vi "Configure Video Trigger.vi"(0 "VISA resource name":refnum<visa-resource-name>, 1 "Wide Video Frequency Width (800E6 Hz)":dbl=800000000.0 format="%^#_9g", 2 "Narrow Video Frequency Center (1E9 Hz)":dbl=1000000000.0 format="%^#_9g", 5 "Minimum Power Level (-20 dB)":i32=-20 format="%^#_9g", 7 "Wide Video Mode (0: In)":u16(ring) items=["In", "Out", "Positive", "Negative"], 9 "Wide Video Frequency Center (1E9 Hz)":dbl=1000000000.0 format="%^#_9g", 11 "error in (no error)":errorcluster, 12 "Narrow Video Mode (0: In)":u16(ring) items=["In", "Out", "Positive", "Negative"], 13 "Narrow Video Frequency Width (13.8E6 Hz)":dbl=13800000.0 format="%^#_9g") -> (4 "VISA resource name out":refnum<visa-resource-name>, 15 "error out":errorcluster)   [LabVIEW 2011, in "Agilent E5052X.lvlib"]
doc: "Configure the video trigger settings for Transient Measurements. \n\n<b>Note: </b>\n\n Be sure to set this first before setting the trigger source to one of the video modes."
uses:
  Agilent E5052X.lvlib
panel:
  # "Wideband Settings"
  # "Narrowband Settings"
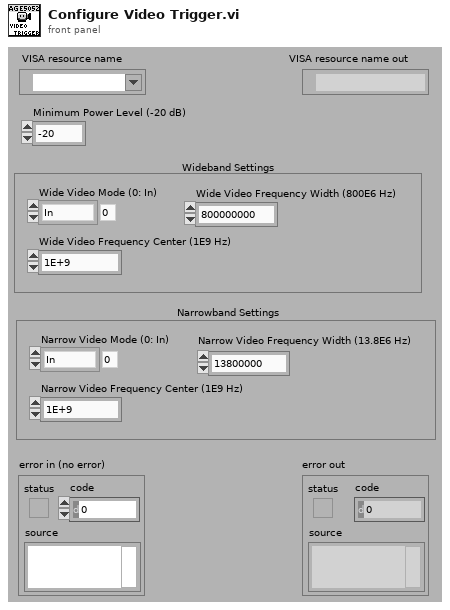
[diagram p1: front panel]
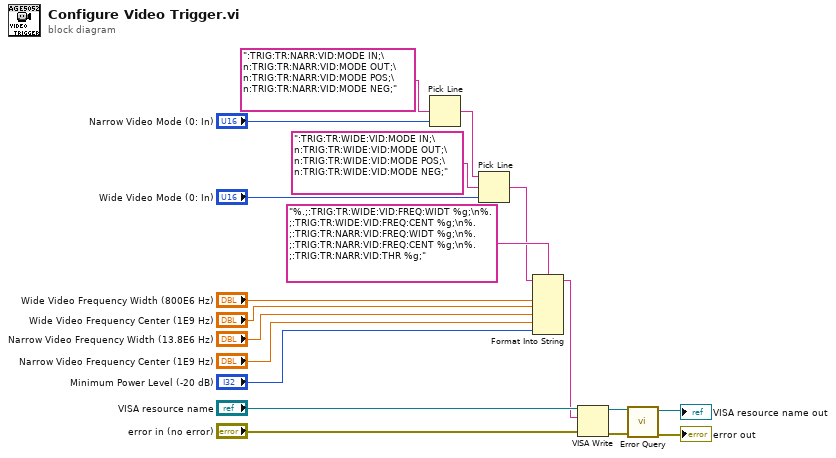
[diagram p0: block diagram]
diagram:
  n1 = Pick Line(multi-line string=":TRIG:TR:NARR:VID:MODE IN;\n:TRIG:TR:NARR:VID:MODE OUT;\n:TRIG:TR:NARR:VID:MODE POS;\n:TRIG:TR:NARR:VID:MODE NEG;", line index="Narrow Video Mode (0: In)") -> (output string=w3:string)  [unwired: 1 in]
  n2 = Pick Line(string ("")=w3, multi-line string=":TRIG:TR:WIDE:VID:MODE IN;\n:TRIG:TR:WIDE:VID:MODE OUT;\n:TRIG:TR:WIDE:VID:MODE POS;\n:TRIG:TR:WIDE:VID:MODE NEG;", line index="Wide Video Mode (0: In)") -> (output string=w2:string)
  n3 = Format Into String(format string="%.;:TRIG:TR:WIDE:VID:FREQ:WIDT %g;\n%.;:TRIG:TR:WIDE:VID:FREQ:CENT %g;\n%.;:TRIG:TR:NARR:VID:FREQ:WIDT %g;\n%.;:TRIG:TR:NARR:VID:FREQ:CENT %g;\n%.;:TRIG:TR:NARR:VID:THR %g;", initial string=w2, "Wide Video Frequency Width (800E6 Hz)", "Wide Video Frequency Center (1E9 Hz)", "Narrow Video Frequency Width (13.8E6 Hz)", "Narrow Video Frequency Center (1E9 Hz)", "Minimum Power Level (-20 dB)") -> (resulting string=w1:string)  [unwired: 1 in, 1 out]
  n4 = VISA Write(VISA resource name="VISA resource name", write buffer=w1, error in (no error)="error in (no error)") -> (VISA resource name out=w12:refnum<visa-resource-name>, error out=w11:errorcluster)  [unwired: 1 out]
  n5 = call "Error Query.vi"("error in (no error)"=w11, "VISA resource name"=w12) -> ("error out"=→"error out":errorcluster, "VISA resource name out"=→"VISA resource name out":refnum<visa-resource-name>)  [unwired: 6 in, 2 out]
